vi "Test - Draw Line - Octant 0.vi"() -> ()   [LabVIEW 2022 SP3, in "Raster.lvlib"]
uses:
  Raster.lvlib
  Point 2D (I32).ctl
  Rectangle Dimensions.ctl
  Utility/Convert Pixels To Picture.vi/d601d993-a776-4dc8-89c7-357d8398c88c.vi
  Utility/Convert Pixels To Picture.vi/7816d0d6-8e4d-41a2-85ac-ed82f1435763.vi
  <vilib>/Utility/High Resolution Relative Seconds.vi
  <vilib>/picture/picture.llb/Draw Unflattened Pixmap.vi
  <vilib>/picture/picture.llb/Draw True-Color Pixmap.vi
  <vilib>/Analysis/baseanly.llb/Mean (DBL).vi
  Utility/Utility.lvlib
  <vilib>/Analysis/NI_AALBase.lvlib
panel:
  out "mean":dbl format="%.1p"
  out "new picture":picture
  out "Pixel Data out":u32[][](array[colorbox])
  # "(0,0)"
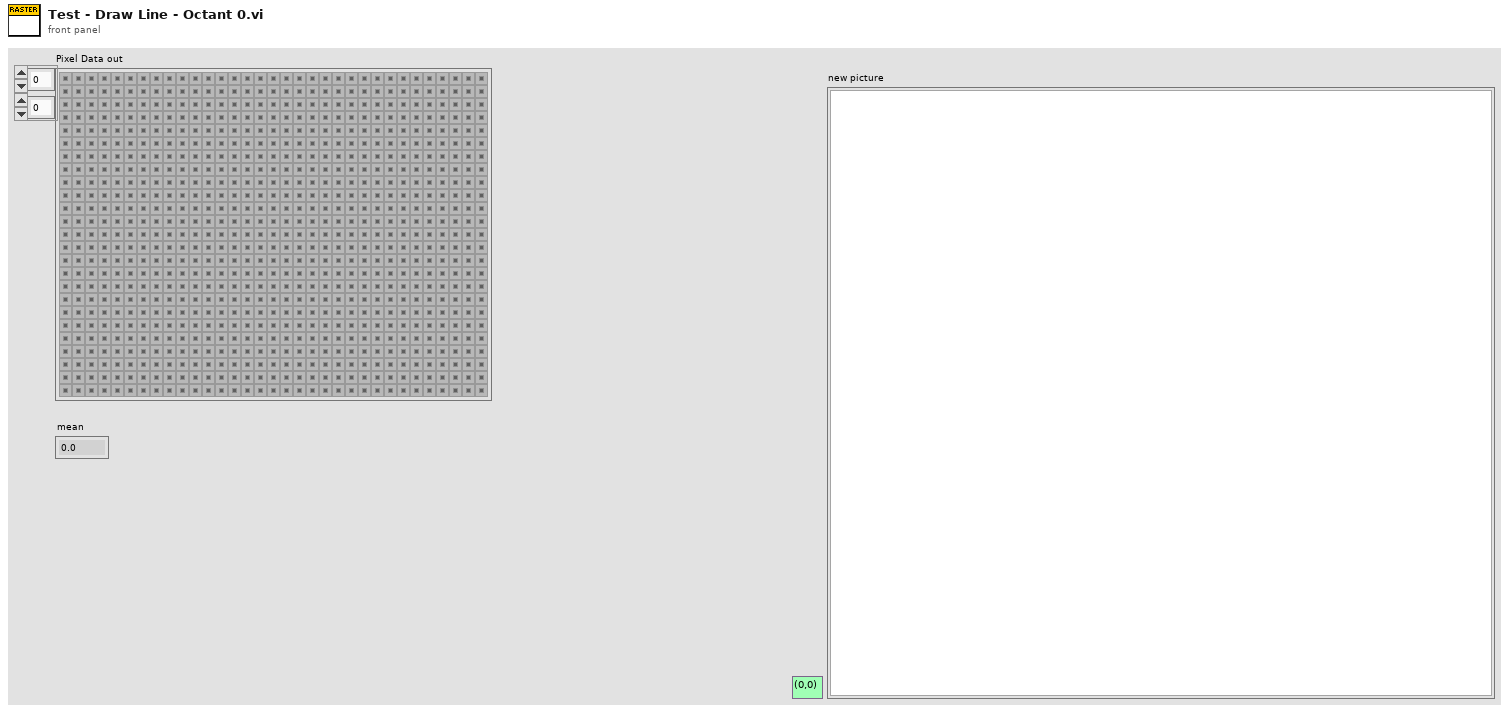
[diagram p1: front panel]
types:
  T1 = typedef "Raster.lvlib/Rectangle Dimensions.ctl" = cluster{"Width":u32, "Height":u32}
  T2 = typedef "Raster.lvlib/Point 2D (I32).ctl" = cluster{"x":i32, "y":i32}
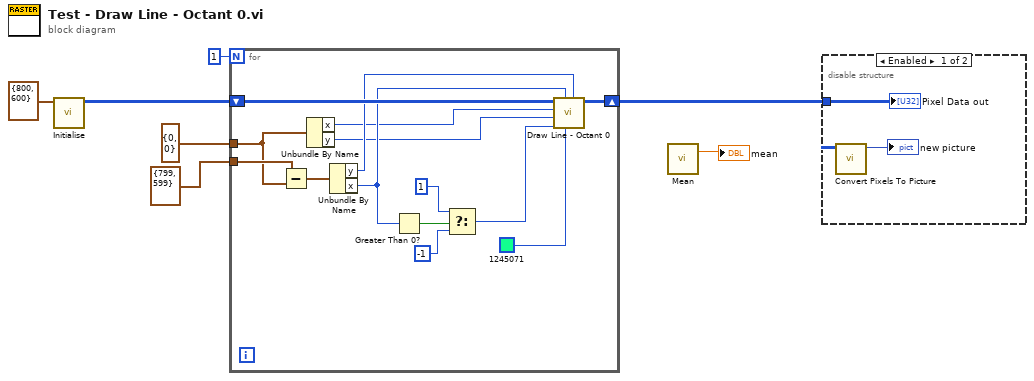
[diagram p0: block diagram]
diagram:
  n1 = call "Initialise.vi"("Screen Dimensions"=T1 {"Width"=800, "Height"=600}) -> ("Pixel Data out"=w6:u32[][])  [unwired: 10 in]
  n2 = for {
    N: 1 -> [_]
    shift-right: [w20] -> w5
    shift-left: w6 -> [w21]
    tunnel: T2 {"x"=0, "y"=0} ("Point 1") -> [w10]
    tunnel: T2 {"x"=799, "y"=599} ("Point 1") -> [w14]
    n3 = Subtract(x=w14, y=w10) -> (x-y=w17:T2)
    n4 = Unbundle By Name(w10) -> ("x"=w9:i32, "y"=w8:i32)
    n5 = Unbundle By Name(w17) -> ("y"=w11:i32, "x"=w12:i32)
    n6 = Greater Than 0?(x=w12) -> (x > 0?=w18:bool)
    n7 = Select(t=1, s=w18, f=-1 ("t")) -> (s? t:f=w13:i32)
    n8 = call "Draw Line - Octant 0.vi"("Delta y"=w11, "Colour"=u32 1245071, "Delta x"=w12, "x Direction"=w13, "Y0"=w8, "X0"=w9, "Pixel Data in"=w21) -> ("Pixel Data out"=w20:u32[][])  [unwired: 4 in]
  }
  n9 = call-poly <vilib>:"Mean.vi"() -> ("mean"=→"mean":dbl)  [unwired: 1 in, 1 out]
  n10 = disable-structure shown="Enabled" {
    disable-tunnel: w5 -> [w22 _]
    frame Enabled {
      n11 = call "Convert Pixels To Picture.vi"("Pixel Data in"=w22) -> ("2D Picture"=→"new picture":picture)  [unwired: 9 in, 1 out]
      "Pixel Data out" <- w22
    }
    frame Disabled {
    }
  }
